vi "Initialize.vi"() -> (3 "Internal Data Out":T1)   [LabVIEW 2025]
uses:
  Internal Data.ctl
  Collision Box.ctl
  <vilib>/picture/picture.llb/imagedata.ctl
types:
  T1 = typedef "Internal Data.ctl" = cluster{"Core":cluster{"Current VI Reference":refnum<vi>, "Close Panel on Exit?":bool}, "Collision Box":T2, "Walls":cluster{"[0]":T3, "[1]":T3, "[2]":T3, "[3]":T3, "[4]":T3, "[5]":T3, "[6]":T3, "[7]":T3, "[8]":T3}, "Floor":T3, "Gates":cluster{"[0]":T3, "[1]":T3, "[2]":T3, "[3]":T3, "[4]":T3, "[5]":T3, "[6]":T3, "[7]":T3, "[8]":T3}, "Gate Condition":bool[], "Level":i32, "Score":i32, "Player Image":T3, "Display Font":cluster{"Font Name:":string, "Size":i16, "Strikeout?":bool, "Italic?":bool, "Underline?":bool, "Outline?":bool, "Shadow?":bool, "Bold?":bool}, "Menu Image":T3, "Menu Button Image":T3, "Menu Selected Image":T3, "Menu Selection":i32, "Player Name":string, "Menu Wall Image":T3}
  T2 = typedef "Collision Box.ctl" = cluster{"left":i16, "top":i16, "right":i16, "bottom":i16}
  T3 = typedef "imagedata.ctl" = cluster{"image type":i32, "image depth":i32, "image":u8[], "mask":u8[], "colors":u32[], "Rectangle":cluster{"left":i16, "top":i16, "right":i16, "bottom":i16}}
  T4 = cluster{"[0]":T3, "[1]":T3, "[2]":T3, "[3]":T3, "[4]":T3, "[5]":T3, "[6]":T3, "[7]":T3, "[8]":T3}
  T5 = cluster{"Font Name:":string, "Size":i16, "Strikeout?":bool, "Italic?":bool, "Underline?":bool, "Outline?":bool, "Shadow?":bool, "Bold?":bool}
  T6 = cluster{"left":i16, "top":i16, "right":i16, "bottom":i16}[]
  T7 = cluster{"Current VI Reference":refnum<vi>, "Close Panel on Exit?":bool}
  T8 = cluster{"left":i16, "top":i16, "right":i16, "bottom":i16}
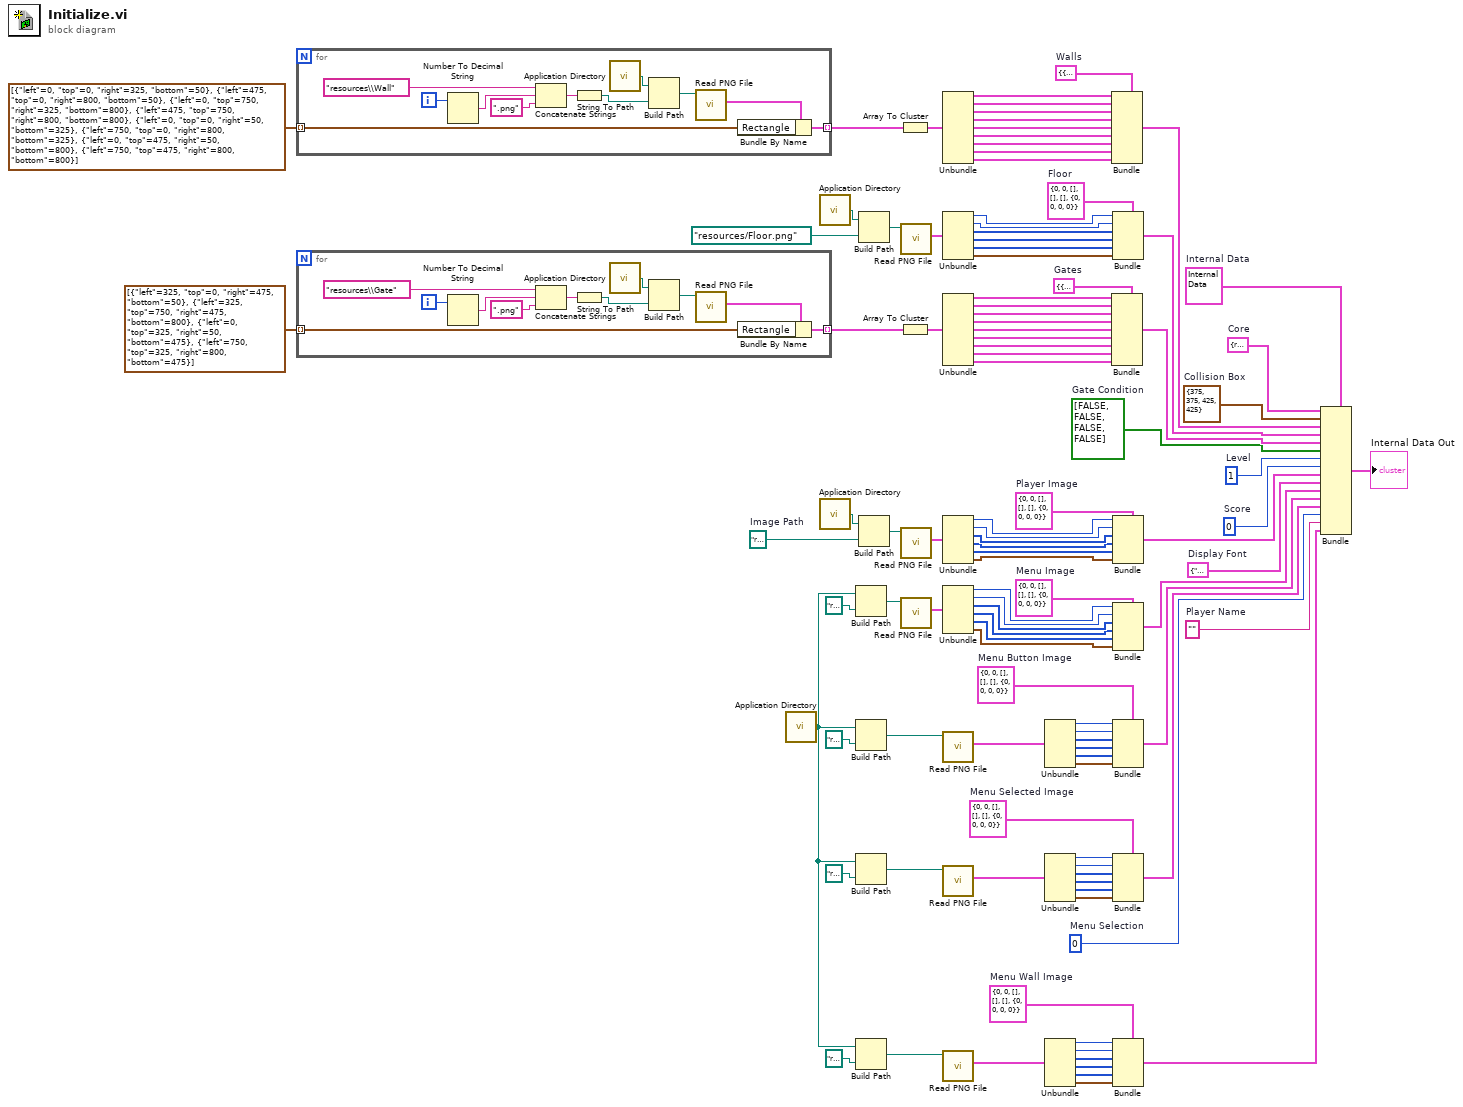
[diagram p0: block diagram]
diagram:
  w7 = T3 {"image type"=0, "image depth"=0, "image"=[], "mask"=[], "colors"=[], "Rectangle"={"left"=0, "top"=0, "right"=0, "bottom"=0}}  # Menu Wall Image
  w16 = T1 {"Core"={"Current VI Reference"=refnum, "Close Panel on Exit?"=FALSE}, "Collision Box"={"left"=0, "top"=0, "right"=0, "bottom"=0}, "Walls"={"[0]"={"image type"=0, "image depth"=0, "image"=[], "mask"=[], "colors"=[], "Rectangle"={"left"=0, "top"=0, "right"=0, "bottom"=0}}, "[1]"={"image type"=0, "image depth"=0, "image"=[], "mask"=[], "colors"=[], "Rectangle"={"left"=0, "top"=0, "right"=0, "bottom"=0}}, "[2]"={"image type"=0, "image depth"=0, "image"=[], "mask"=[], "colors"=[], "Rectangle"={"left"=0, "top"=0, "right"=0, "bottom"=0}}, "[3]"={"image type"=0, "image depth"=0, "image"=[], "mask"=[], "colors"=[], "Rectangle"={"left"=0, "top"=0, "right"=0, "bottom"=0}}, "[4]"={"image type"=0, "image depth"=0, "image"=[], "mask"=[], "colors"=[], "Rectangle"={"left"=0, "top"=0, "right"=0, "bottom"=0}}, "[5]"={"image type"=0, "image depth"=0, "image"=[], "mask"=[], "colors"=[], "Rectangle"={"left"=0, "top"=0, "right"=0, "bottom"=0}}, "[6]"={"image type"=0, "image depth"=0, "image"=[], "mask"=[], "colors"=[], "Rectangle"={"left"=0, "top"=0, "right"=0, "bottom"=0}}, "[7]"={"image type"=0, "image depth"=0, "image"=[], "mask"=[], "colors"=[], "Rectangle"={"left"=0, "top"=0, "right"=0, "bottom"=0}}, "[8]"={"image type"=0, "image depth"=0, "image"=[], "mask"=[], "colors"=[], "Rectangle"={"left"=0, "top"=0, "right"=0, "bottom"=0}}}, "Floor"={"image type"=0, "image depth"=0, "image"=[], "mask"=[], "colors"=[], "Rectangle"={"left"=0, "top"=0, "right"=0, "bottom"=0}}, "Gates"={"[0]"={"image type"=0, "image depth"=0, "image"=[], "mask"=[], "colors"=[], "Rectangle"={"left"=0, "top"=0, "right"=0, "bottom"=0}}, "[1]"={"image type"=0, "image depth"=0, "image"=[], "mask"=[], "colors"=[], "Rectangle"={"left"=0, "top"=0, "right"=0, "bottom"=0}}, "[2]"={"image type"=0, "image depth"=0, "image"=[], "mask"=[], "colors"=[], "Rectangle"={"left"=0, "top"=0, "right"=0, "bottom"=0}}, "[3]"={"image type"=0, "image depth"=0, "image"=[], "mask"=[], "colors"=[], "Rectangle"={"left"=0, "top"=0, "right"=0, "bottom"=0}}, "[4]"={"image type"=0, "image depth"=0, "image"=[], "mask"=[], "colors"=[], "Rectangle"={"left"=0, "top"=0, "right"=0, "bottom"=0}}, "[5]"={"image type"=0, "image depth"=0, "image"=[], "mask"=[], "colors"=[], "Rectangle"={"left"=0, "top"=0, "right"=0, "bottom"=0}}, "[6]"={"image type"=0, "image depth"=0, "image"=[], "mask"=[], "colors"=[], "Rectangle"={"left"=0, "top"=0, "right"=0, "bottom"=0}}, "[7]"={"image type"=0, "image depth"=0, "image"=[], "mask"=[], "colors"=[], "Rectangle"={"left"=0, "top"=0, "right"=0, "bottom"=0}}, "[8]"={"image type"=0, "image depth"=0, "image"=[], "mask"=[], "colors"=[], "Rectangle"={"left"=0, "top"=0, "right"=0, "bottom"=0}}}, "Gate Condition"=[], "Level"=0, "Score"=0, "Player Image"={"image type"=0, "image depth"=0, "image"=[], "mask"=[], "colors"=[], "Rectangle"={"left"=0, "top"=0, "right"=0, "bottom"=0}}, "Display Font"={"Font Name:"="", "Size"=0, "Strikeout?"=FALSE, "Italic?"=FALSE, "Underline?"=FALSE, "Outline?"=FALSE, "Shadow?"=FALSE, "Bold?"=FALSE}, "Menu Image"={"image type"=0, "image depth"=0, "image"=[], "mask"=[], "colors"=[], "Rectangle"={"left"=0, "top"=0, "right"=0, "bottom"=0}}, "Menu Button Image"={"image type"=0, "image depth"=0, "image"=[], "mask"=[], "colors"=[], "Rectangle"={"left"=0, "top"=0, "right"=0, "bottom"=0}}, "Menu Selected Image"={"image type"=0, "image depth"=0, "image"=[], "mask"=[], "colors"=[], "Rectangle"={"left"=0, "top"=0, "right"=0, "bottom"=0}}, "Menu Selection"=0, "Player Name"="", "Menu Wall Image"={"image type"=0, "image depth"=0, "image"=[], "mask"=[], "colors"=[], "Rectangle"={"left"=0, "top"=0, "right"=0, "bottom"=0}}}  # Internal Data
  w17 = ""  # Player Name
  w18 = 0  # Menu Selection
  w21 = T3 {"image type"=0, "image depth"=0, "image"=[], "mask"=[], "colors"=[], "Rectangle"={"left"=0, "top"=0, "right"=0, "bottom"=0}}  # Menu Selected Image
  w38 = T3 {"image type"=0, "image depth"=0, "image"=[], "mask"=[], "colors"=[], "Rectangle"={"left"=0, "top"=0, "right"=0, "bottom"=0}}  # Menu Button Image
  w1 = T3 {"image type"=0, "image depth"=0, "image"=[], "mask"=[], "colors"=[], "Rectangle"={"left"=0, "top"=0, "right"=0, "bottom"=0}}  # Menu Image
  w59 = T3 {"image type"=0, "image depth"=0, "image"=[], "mask"=[], "colors"=[], "Rectangle"={"left"=0, "top"=0, "right"=0, "bottom"=0}}  # Floor
  w67 = T3 {"image type"=0, "image depth"=0, "image"=[], "mask"=[], "colors"=[], "Rectangle"={"left"=0, "top"=0, "right"=0, "bottom"=0}}  # Player Image
  w70 = T4 {"[0]"={"image type"=0, "image depth"=0, "image"=[], "mask"=[], "colors"=[], "Rectangle"={"left"=0, "top"=0, "right"=0, "bottom"=0}}, "[1]"={"image type"=0, "image depth"=0, "image"=[], "mask"=[], "colors"=[], "Rectangle"={"left"=0, "top"=0, "right"=0, "bottom"=0}}, "[2]"={"image type"=0, "image depth"=0, "image"=[], "mask"=[], "colors"=[], "Rectangle"={"left"=0, "top"=0, "right"=0, "bottom"=0}}, "[3]"={"image type"=0, "image depth"=0, "image"=[], "mask"=[], "colors"=[], "Rectangle"={"left"=0, "top"=0, "right"=0, "bottom"=0}}, "[4]"={"image type"=0, "image depth"=0, "image"=[], "mask"=[], "colors"=[], "Rectangle"={"left"=0, "top"=0, "right"=0, "bottom"=0}}, "[5]"={"image type"=0, "image depth"=0, "image"=[], "mask"=[], "colors"=[], "Rectangle"={"left"=0, "top"=0, "right"=0, "bottom"=0}}, "[6]"={"image type"=0, "image depth"=0, "image"=[], "mask"=[], "colors"=[], "Rectangle"={"left"=0, "top"=0, "right"=0, "bottom"=0}}, "[7]"={"image type"=0, "image depth"=0, "image"=[], "mask"=[], "colors"=[], "Rectangle"={"left"=0, "top"=0, "right"=0, "bottom"=0}}, "[8]"={"image type"=0, "image depth"=0, "image"=[], "mask"=[], "colors"=[], "Rectangle"={"left"=0, "top"=0, "right"=0, "bottom"=0}}}  # Gates
  w92 = T4 {"[0]"={"image type"=0, "image depth"=0, "image"=[], "mask"=[], "colors"=[], "Rectangle"={"left"=0, "top"=0, "right"=0, "bottom"=0}}, "[1]"={"image type"=0, "image depth"=0, "image"=[], "mask"=[], "colors"=[], "Rectangle"={"left"=0, "top"=0, "right"=0, "bottom"=0}}, "[2]"={"image type"=0, "image depth"=0, "image"=[], "mask"=[], "colors"=[], "Rectangle"={"left"=0, "top"=0, "right"=0, "bottom"=0}}, "[3]"={"image type"=0, "image depth"=0, "image"=[], "mask"=[], "colors"=[], "Rectangle"={"left"=0, "top"=0, "right"=0, "bottom"=0}}, "[4]"={"image type"=0, "image depth"=0, "image"=[], "mask"=[], "colors"=[], "Rectangle"={"left"=0, "top"=0, "right"=0, "bottom"=0}}, "[5]"={"image type"=0, "image depth"=0, "image"=[], "mask"=[], "colors"=[], "Rectangle"={"left"=0, "top"=0, "right"=0, "bottom"=0}}, "[6]"={"image type"=0, "image depth"=0, "image"=[], "mask"=[], "colors"=[], "Rectangle"={"left"=0, "top"=0, "right"=0, "bottom"=0}}, "[7]"={"image type"=0, "image depth"=0, "image"=[], "mask"=[], "colors"=[], "Rectangle"={"left"=0, "top"=0, "right"=0, "bottom"=0}}, "[8]"={"image type"=0, "image depth"=0, "image"=[], "mask"=[], "colors"=[], "Rectangle"={"left"=0, "top"=0, "right"=0, "bottom"=0}}}  # Walls
  w103 = T5 {"Font Name:"="Font", "Size"=24, "Strikeout?"=FALSE, "Italic?"=FALSE, "Underline?"=FALSE, "Outline?"=FALSE, "Shadow?"=FALSE, "Bold?"=TRUE}  # Display Font
  w95 = path "resources/Down0.png"  # Image Path
  w104 = T2 {"left"=375, "top"=375, "right"=425, "bottom"=425}  # Collision Box
  w105 = 0  # Score
  w106 = 1  # Level
  w2 = bool[] [FALSE, FALSE, FALSE, FALSE]  # Gate Condition
  w107 = T7 {"Current VI Reference"=refnum, "Close Panel on Exit?"=FALSE}  # Core
  n1 = for {
    tunnel: [w115] -> w94 mode=indexing
    tunnel: T6 [{"left"=0, "top"=0, "right"=325, "bottom"=50}, {"left"=475, "top"=0, "right"=800, "bottom"=50}, {"left"=0, "top"=750, "right"=325, "bottom"=800}, {"left"=475, "top"=750, "right"=800, "bottom"=800}, {"left"=0, "top"=0, "right"=50, "bottom"=325}, {"left"=750, "top"=0, "right"=800, "bottom"=325}, {"left"=0, "top"=475, "right"=50, "bottom"=800}, {"left"=750, "top"=475, "right"=800, "bottom"=800}] -> [w108] mode=indexing
    i -> [w109]
    n2 = Number To Decimal String(number=w109) -> (decimal integer string=w111:string)  [unwired: 1 in]
    n3 = Concatenate Strings("resources\\Wall" ("string"), w111, ".png" ("string")) -> (w113:string)
    n4 = String To Path(string=w113) -> (path=w114:path)
    n5 = call <vilib>:"Application Directory.vi"() -> ("Application Directory"=w118:path)
    n6 = Build Path(base path=w118, name or relative path=w114) -> (appended path=w117:path)
    n7 = call <vilib>:"Read PNG File.vi"("path to PNG file"=w117) -> ("image data"=w116:T3)  [unwired: 8 in, 2 out]
    n8 = Bundle By Name(cluster=w116, "Rectangle"=w108) -> (w115:T3)
  }
  n9 = for {
    tunnel: [w126] -> w81 mode=indexing
    tunnel: T6 [{"left"=325, "top"=0, "right"=475, "bottom"=50}, {"left"=325, "top"=750, "right"=475, "bottom"=800}, {"left"=0, "top"=325, "right"=50, "bottom"=475}, {"left"=750, "top"=325, "right"=800, "bottom"=475}] -> [w119] mode=indexing
    i -> [w120]
    n10 = Number To Decimal String(number=w120) -> (decimal integer string=w122:string)  [unwired: 1 in]
    n11 = Concatenate Strings("resources\\Gate" ("string"), w122, ".png" ("string")) -> (w124:string)
    n12 = String To Path(string=w124) -> (path=w125:path)
    n13 = call <vilib>:"Application Directory.vi"() -> ("Application Directory"=w129:path)
    n14 = Build Path(base path=w129, name or relative path=w125) -> (appended path=w128:path)
    n15 = call <vilib>:"Read PNG File.vi"("path to PNG file"=w128) -> ("image data"=w127:T3)  [unwired: 8 in, 2 out]
    n16 = Bundle By Name(cluster=w127, "Rectangle"=w119) -> (w126:T3)
  }
  n17 = call <vilib>:"Application Directory.vi"() -> ("Application Directory"=w5:path)
  n18 = call <vilib>:"Application Directory.vi"() -> ("Application Directory"=w102:path)
  n19 = call <vilib>:"Application Directory.vi"() -> ("Application Directory"=w97:path)
  n20 = Build Path(base path=w5, name or relative path=path "resources/Menu.png") -> (appended path=w49:path)
  n21 = Build Path(base path=w5, name or relative path=path "resources/Menu_Button.png") -> (appended path=w39:path)
  n22 = Build Path(base path=w5, name or relative path=path "resources/Menu_Button_Selected.png") -> (appended path=w22:path)
  n23 = Build Path(base path=w5, name or relative path=path "resources/Wall.png") -> (appended path=w14:path)
  n24 = Build Path(base path=w102, name or relative path=path "resources/Floor.png") -> (appended path=w101:path)
  n25 = Build Path(base path=w97, name or relative path=w95) -> (appended path=w96:path)
  n26 = Array To Cluster(array=w94) -> (cluster=w93:T4)
  n27 = Array To Cluster(array=w81) -> (cluster=w71:T4)
  n28 = call <vilib>:"Read PNG File.vi"("path to PNG file"=w101) -> ("image data"=w52:T3)  [unwired: 8 in, 2 out]
  n29 = call <vilib>:"Read PNG File.vi"("path to PNG file"=w96) -> ("image data"=w68:T3)  [unwired: 8 in, 2 out]
  n30 = call <vilib>:"Read PNG File.vi"("path to PNG file"=w49) -> ("image data"=w43:T3)  [unwired: 8 in, 2 out]
  n31 = Unbundle(w93) -> ("[0]"=w90:T3, "[1]"=w89:T3, "[2]"=w88:T3, "[3]"=w87:T3, "[4]"=w86:T3, "[5]"=w85:T3, "[6]"=w84:T3, "[7]"=w83:T3, "[8]"=w82:T3)
  n32 = Unbundle(w52) -> ("image type"=w58:i32, "image depth"=w57:i32, "image"=w56:u8[], "mask"=w55:u8[], "colors"=w54:u32[], "Rectangle"=w53:T8)
  n33 = Unbundle(w71) -> ("[0]"=w80:T3, "[1]"=w79:T3, "[2]"=w78:T3, "[3]"=w77:T3, "[4]"=w76:T3, "[5]"=w75:T3, "[6]"=w74:T3, "[7]"=w73:T3, "[8]"=w72:T3)
  n34 = Unbundle(w68) -> ("image type"=w66:i32, "image depth"=w65:i32, "image"=w64:u8[], "mask"=w63:u8[], "colors"=w62:u32[], "Rectangle"=w61:T8)
  n35 = Unbundle(w43) -> ("image type"=w48:i32, "image depth"=w47:i32, "image"=w46:u8[], "mask"=w45:u8[], "colors"=w44:u32[], "Rectangle"=w42:T8)
  n36 = call <vilib>:"Read PNG File.vi"("path to PNG file"=w39) -> ("image data"=w31:T3)  [unwired: 8 in, 2 out]
  n37 = call <vilib>:"Read PNG File.vi"("path to PNG file"=w22) -> ("image data"=w20:T3)  [unwired: 8 in, 2 out]
  n38 = call <vilib>:"Read PNG File.vi"("path to PNG file"=w14) -> ("image data"=w15:T3)  [unwired: 8 in, 2 out]
  n39 = Unbundle(w31) -> ("image type"=w37:i32, "image depth"=w36:i32, "image"=w35:u8[], "mask"=w34:u8[], "colors"=w33:u32[], "Rectangle"=w32:T8)
  n40 = Unbundle(w20) -> ("image type"=w28:i32, "image depth"=w27:i32, "image"=w26:u8[], "mask"=w25:u8[], "colors"=w24:u32[], "Rectangle"=w23:T8)
  n41 = Unbundle(w15) -> ("image type"=w8:i32, "image depth"=w9:i32, "image"=w10:u8[], "mask"=w11:u8[], "colors"=w12:u32[], "Rectangle"=w13:T8)
  n42 = Bundle(cluster=w92, "[0]"=w90, "[1]"=w89, "[2]"=w88, "[3]"=w87, "[4]"=w86, "[5]"=w85, "[6]"=w84, "[7]"=w83, "[8]"=w82) -> (w91:T4)
  n43 = Bundle(cluster=w70, "[0]"=w80, "[1]"=w79, "[2]"=w78, "[3]"=w77, "[4]"=w76, "[5]"=w75, "[6]"=w74, "[7]"=w73, "[8]"=w72) -> (w69:T4)
  n44 = Bundle(cluster=w59, "image type"=w58, "image depth"=w57, "image"=w56, "mask"=w55, "colors"=w54, "Rectangle"=w53) -> (w51:T3)
  n45 = Bundle(cluster=w67, "image type"=w66, "image depth"=w65, "image"=w64, "mask"=w63, "colors"=w62, "Rectangle"=w61) -> (w60:T3)
  n46 = Bundle(cluster=w1, "image type"=w48, "image depth"=w47, "image"=w46, "mask"=w45, "colors"=w44, "Rectangle"=w42) -> (w41:T3)
  n47 = Bundle(cluster=w38, "image type"=w37, "image depth"=w36, "image"=w35, "mask"=w34, "colors"=w33, "Rectangle"=w32) -> (w30:T3)
  n48 = Bundle(cluster=w21, "image type"=w28, "image depth"=w27, "image"=w26, "mask"=w25, "colors"=w24, "Rectangle"=w23) -> (w19:T3)
  n49 = Bundle(cluster=w7, "image type"=w8, "image depth"=w9, "image"=w10, "mask"=w11, "colors"=w12, "Rectangle"=w13) -> (w4:T3)
  n50 = Bundle "Bundle"(cluster=w16, "Core"=w107, "Collision Box"=w104, "Walls"=w91, "Floor"=w51, "Gates"=w69, "Gate Condition"=w2, "Level"=w106, "Score"=w105, "Player Image"=w60, "Display Font"=w103, "Menu Image"=w41, "Menu Button Image"=w30, "Menu Selected Image"=w19, "Menu Selection"=w18, "Player Name"=w17, "Menu Wall Image"=w4) -> (→"Internal Data Out":T1)
